vi "Source Overvoltage Protection.vi"(0 "VISA resource name":refnum<visa-resource-name>, 5 "Node In":string, 7 "Maximum Source Voltage":sgl, 11 "error in (no error)":errorcluster) -> (4 "VISA resource name out":refnum<visa-resource-name>, 6 "Node Out":string, 15 "error out":errorcluster)   [LabVIEW 2009, in "Keithley 2600 Series.lvlib"]
doc: "This VI controls the overvoltage protection limit. Setting this attribute to zero disables overvoltage protection. When this attribute is set to a nonzero value, the SMU will limit the voltage on the force leads to the value specified by this attribute. This feature is exclusive to the 2657A line of instruments.\n\n<b>Functions and Attributes Used</b>\nsmux.source.protectv"
uses:
  <instrlib>/Keithley 2600 Series/Private/GlobalVariables.vi
  <instrlib>/Keithley 2600 Series/Keithley 2600 Series.lvlib
panel:
  # "(c) 2011 Keithley Instruments, Inc.  ALL RIGHTS RESERVED."
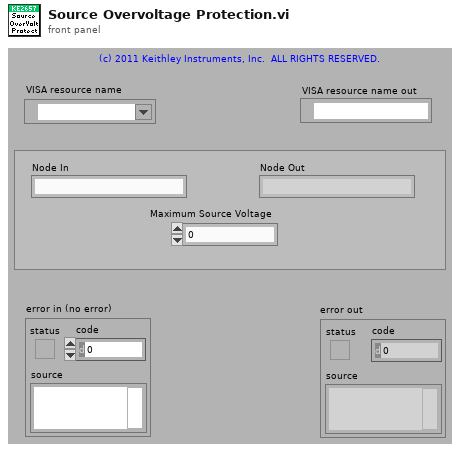
[diagram p1: front panel]
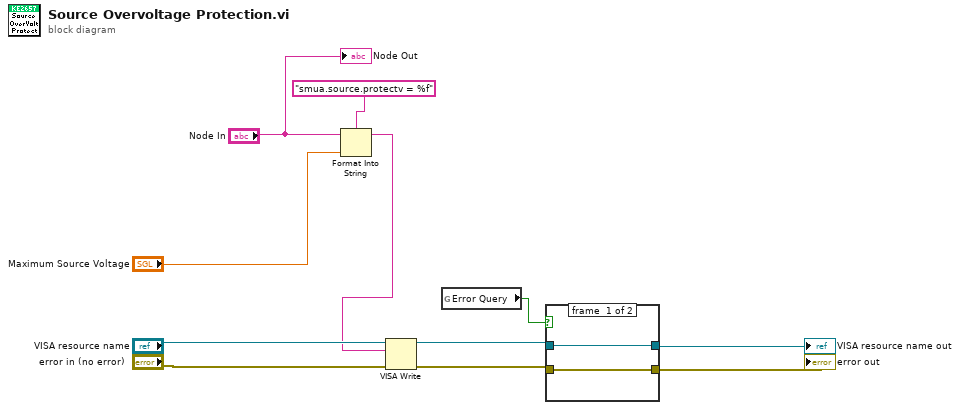
[diagram p0: block diagram]
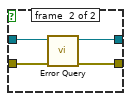
[diagram p2: hidden frame]
diagram:
  n1 = Format Into String(format string="smua.source.protectv = %f", initial string="Node In", "Maximum Source Voltage") -> (resulting string=w3:string)  [unwired: 1 in, 1 out]
  n2 = VISA Write(VISA resource name="VISA resource name", write buffer=w3, error in (no error)="error in (no error)") -> (VISA resource name out=w10:refnum<visa-resource-name>, error out=w9:errorcluster)  [unwired: 1 out]
  n3 = global read "GlobalVariables.vi" "Error Query"() -> (w11:bool)
  n4 = case shown="True" w11 {
    tunnel: w10 -> [w13 w17]
    tunnel: w9 -> [w12 w16]
    tunnel: [w13 w15] -> w2
    tunnel: [w12 w14] -> w1
    frame #0 {
    }
    frame #1 {
      n5 = call <instrlib>:"Error Query.vi"("error in (no error)"=w16, "VISA resource name"=w17) -> ("error out"=w14:errorcluster, "VISA resource name out"=w15:refnum<visa-resource-name>)  [unwired: 8 out]
    }
  }
  "VISA resource name out" <- w2
  "error out" <- w1
  "Node Out" <- "Node In"
